vi "Measurements.vi"(3 "error in":errorcluster {"code" format="%.0x"}, 4 "Measurements":T3, 5 "instrument handle":refnum<k15>, 6 "Enabled Channels cluster":T2) -> (0 "error out":errorcluster {"code" format="%.0x"}, 1 "Measurement results":T1 {"result  3" format="%.2f"; "result  2" format="%.2f"; "result" format="%.2f"}, 2 "instrument handle out":refnum<k15>)   [LabVIEW 2011]
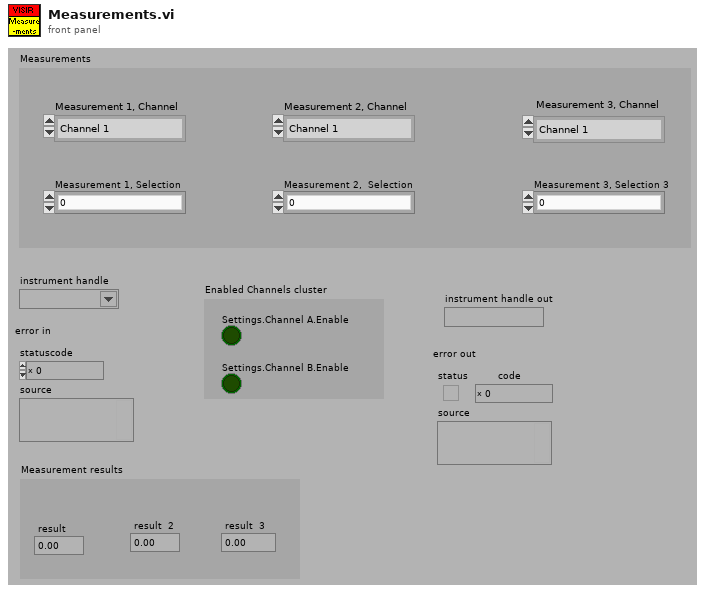
[diagram p1: front panel]
types:
  T1 = cluster{" result ":dbl, " result  2":dbl, " result  3":dbl}
  T2 = cluster{"Settings.Channel A.Enable":bool, "Settings.Channel B.Enable":bool}
  T3 = cluster{"Measurement 1, Channel":enum8{"Channel 1", "Channel 2", "Channel 3", "Channel 4"}, "Measurement 1, Selection":u16, "Measurement 2, Channel":enum8{"Channel 1", "Channel 2", "Channel 3", "Channel 4"}, "Measurement 2,  Selection":u16, "Measurement 3, Channel":enum8{"Channel 1", "Channel 2", "Channel 3", "Channel 4"}, "Measurement 3, Selection 3":u16}
  T4 = enum8{"Channel 1", "Channel 2", "Channel 3", "Channel 4"}
  T5 = cluster{"result":dbl, "result":dbl, "result":dbl}
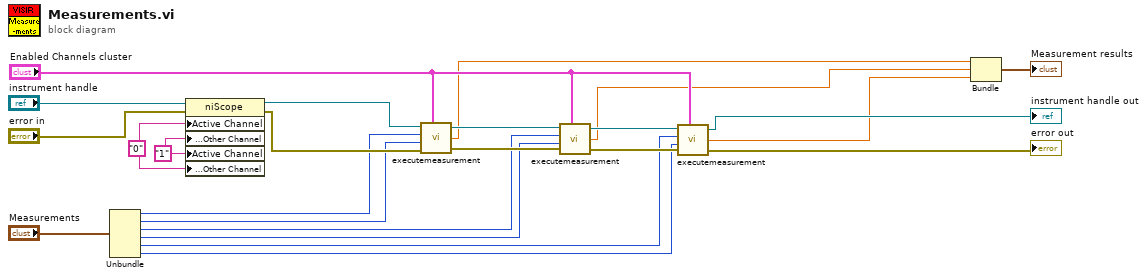
[diagram p0: block diagram]
diagram:
  w24 = "0"
  w23 = "1"
  n1 = Unbundle("Measurements") -> ("Measurement 1, Channel"=w16:T4, "Measurement 1, Selection"=w17:u16, "Measurement 2, Channel"=w13:T4, "Measurement 2,  Selection"=w12:u16, "Measurement 3, Channel"=w6:T4, "Measurement 3, Selection 3"=w5:u16)
  n2 = property class="niScope"(reference="instrument handle", error in="error in", "Active Channel"=w24, "Waveform Measurement:Other Channel"=w23, "Active Channel"=w23, "Waveform Measurement:Other Channel"=w24) -> (reference out=w19:refnum<k15>, error out=w18:errorcluster)
  n3 = call "executemeasurement.vi"("instrument handle in"=w19, "Measurement Channel"=w16, "Measurement  Selection"=w17, "Error In"=w18, "Enabled Channels cluster"="Enabled Channels cluster") -> ("Instrument handle out"=w15:refnum<k15>, "result"=w4:dbl, "Error Out"=w14:errorcluster)
  n4 = call "executemeasurement.vi"("instrument handle in"=w15, "Measurement Channel"=w13, "Measurement  Selection"=w12, "Error In"=w14, "Enabled Channels cluster"="Enabled Channels cluster") -> ("Instrument handle out"=w10:refnum<k15>, "result"=w3:dbl, "Error Out"=w9:errorcluster)
  n5 = call "executemeasurement.vi"("instrument handle in"=w10, "Measurement Channel"=w6, "Measurement  Selection"=w5, "Error In"=w9, "Enabled Channels cluster"="Enabled Channels cluster") -> ("Instrument handle out"=→"instrument handle out":refnum<k15>, "result"=w2:dbl, "Error Out"=→"error out":errorcluster)
  n6 = Bundle("result"=w4, "result"=w3, "result"=w2) -> (→"Measurement results":T5)  [unwired: 1 in]
